vi "U8Array_to_U32Array.vi"(10 "U8":u8[](array[numeric])) -> (2 "U32":u32[](array[numeric]))   [LabVIEW 2013, in "NI_SHA-256(2013).lvlib" / "NI_SHA-256.lvclass"]
uses:
  NI_SHA-256.lvclass
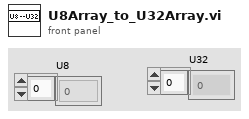
[diagram p1: front panel]
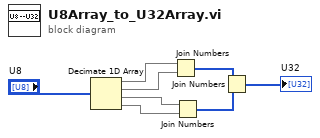
[diagram p0: block diagram]
diagram:
  n1 = Decimate 1D Array("U8") -> (w4:u8[], w3:u8[], w2:u8[], w1:u8[])
  n2 = Join Numbers(hi=w4, lo=w3) -> ((hi.lo)=w8:u16[])
  n3 = Join Numbers(hi=w2, lo=w1) -> ((hi.lo)=w7:u16[])
  n4 = Join Numbers(hi=w8, lo=w7) -> ((hi.lo)=→"U32":u32[])
